vi "bool 2d array to uint array.vi"(1 "bool [] []":bool[][](array[boolean])) -> (0 "integer []":u32[](array[numeric]))   [LabVIEW 2021]
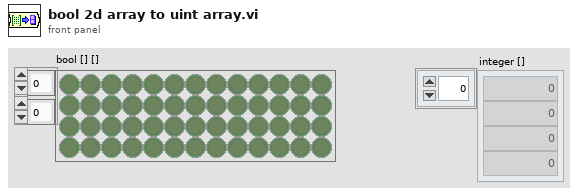
[diagram p1: front panel]
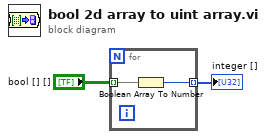
[diagram p0: block diagram]
diagram:
  n1 = for {
    tunnel: "bool [] []" -> [w4] mode=indexing
    tunnel: [w3] -> w1 mode=indexing
    n2 = Boolean Array To Number(Boolean array=w4) -> (number=w3:u32)
  }
  "integer []" <- w1
